vi "Configure Temperature.vi"(8 "error in (no error)":errorcluster, 9 "Resistor Channel":i32, 10 "temperature (C)":dbl=25.0, 11 "PRM in":refnum<class "PRM.lvclass">) -> (0 "error out":errorcluster, 3 "PRM out":refnum<class "PRM.lvclass">)   [LabVIEW 2019]
uses:
  <instrlib>/ni272xReferenceVIs/ni272xReferenceVIs.llb/ni272x Write Resistance 1Chan 1Samp.vi
  Library/PRM.lvclass
  builds/Instruments/Instruments.lvlibp/Library/Instruments.lvclass
  builds/Instruments/Instruments.lvlibp/Private/Polymorphic/Special/Event from String.vi
  builds/Instruments/Instruments.lvlibp
  C:/Users/Public/Documents/Development/builds/Instruments/Instruments.lvlibp/Library/Instruments.lvclass
  C:/Users/Public/Documents/Development/builds/Tools/Config.lvlibp/Config.lvclass
  C:/Users/Public/Documents/Development/builds/Engine/Engine.lvlibp/Project/Engine.lvclass
  C:/Users/Public/Documents/Development/builds/Engine/State Actor.lvlibp/Library/State Actor.lvclass
  C:/Users/Public/Documents/Development/builds/Engine/Panel Manager.lvlibp/Panel Actor/Panel Actor.lvclass
  C:/Users/Public/Documents/Development/builds/Engine/Monitored Actor.lvlibp/Monitored Actor/Monitored Actor/Monitored Actor.lvclass
  C:/Users/Public/Documents/Development/builds/Engine/Actor Framework.lvlibp/1abvi3w/vi.lib/ActorFramework/Actor/Actor.lvclass
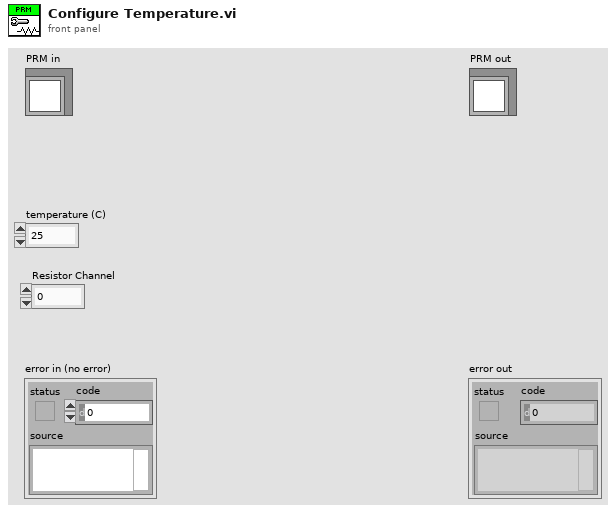
[diagram p1: front panel]
types:
  T1 = cluster{"Timestamp":timestamp, "Description":string, "Data":string}
  T2 = typedef "ni272x Reference.ctl" = refnum<k20>
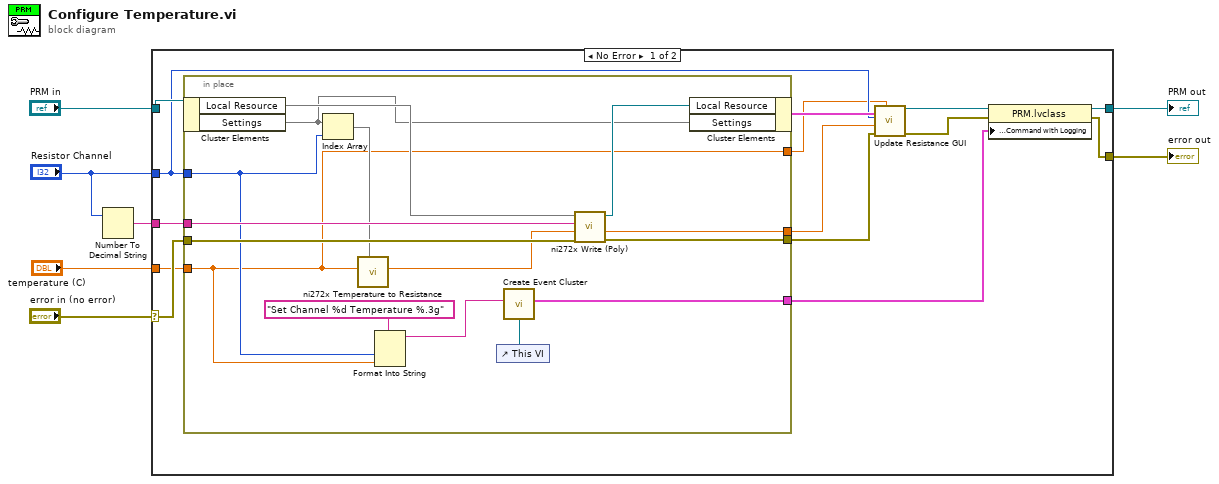
[diagram p0: block diagram]
diagram:
  n1 = Number To Decimal String(number="Resistor Channel") -> (decimal integer string=w1:string)  [unwired: 1 in]
  n2 = case shown="No Error" "error in (no error)" {
    selector: "error in (no error)" -> [w19 w38]
    tunnel: [w9 w38] -> w6
    tunnel: [w12 w37] -> w4
    tunnel: "PRM in" -> [w20 w37]
    tunnel: w1 -> [w21 _]
    tunnel: "temperature (C)" -> [w18 _]
    tunnel: "Resistor Channel" -> [w16 _]
    frame No Error {
      n3 = in-place {
        in-place-border: w21 -> [w33]
        in-place-border: w19 -> [w34]
        in-place-border: [w30] -> w14
        in-place-border: w18 -> [w22]
        in-place-border: w16 -> [w25]
        in-place-border: [w29] -> w15
        in-place-border: [w24] -> w11
        in-place-border: [w22] -> w8
        n4 = in-place-cluster #1(w20) -> ("Local Resource"=w36, "Settings"=w31)
        n5 = Index Array(array=w31, index=w25) -> (element=w32)
        n6 = call <instrlib>:"ni272x Temperature to Resistance.vi"("Callendar-Van Dusen RTD parameters"=w32, "temperature (degrees Celsius)"=w22) -> ("resistance (ohms)"=w23:dbl)  [unwired: 9 in]
        n7 = Format Into String(format string="Set Channel %d Temperature %.3g", w25, w22) -> (resulting string=w26:string)  [unwired: 2 in, 1 out]
        n8 = control-ref of="This VI"() -> (w28:refnum<vi>)
        n9 = call-poly "Create Event Cluster.vi"("Value"=w26, "VI Refnum"=w28) -> ("Event Data"=w24:T1)  [unwired: 9 in]
        n10 = call-poly <instrlib>:"ni272x Write (Poly).vi"("error in (no error)"=w34, "requested resistance (ohms)"=w23, "resistor channel"=w33, "instrument handle"=w36) -> ("error out"=w30:errorcluster, "coerced resistance (ohms)"=w29:dbl, "instrument handle out"=w35:T2)  [unwired: 5 out]
        n11 = in-place-cluster #1("Local Resource"=w35, "Settings"=w31) -> (w17:cluster{})
      }
      n12 = call "Update Resistance GUI.vi"("temperature"=w8, "error in (no error)"=w14, "resistance"=w15, "Resistor Channel"=w16, "PRM in"=w17) -> ("error out"=w10:errorcluster, "PRM out"=w13:refnum<class "PRM.lvclass">)  [unwired: 5 in]
      n13 = property class="PRM.lvclass"(reference=w13, error in=w10, "Accessors:Logging:Command with Logging"=w11) -> (reference out=w12:refnum<class "PRM.lvclass">, error out=w9:errorcluster)
    }
    frame Error {
    }
  }
  "error out" <- w6
  "PRM out" <- w4
